vi "通道数对话框.vi"(8 "error in (no error)":errorcluster) -> (0 "error out":errorcluster)   [LabVIEW 2015]
uses:
  Global/SeverGlobal.vi
panel:
  in  "OK":bool
  in  "Channel count":enum16{"64X4", "128X4"}(ring)=enum."128X4"
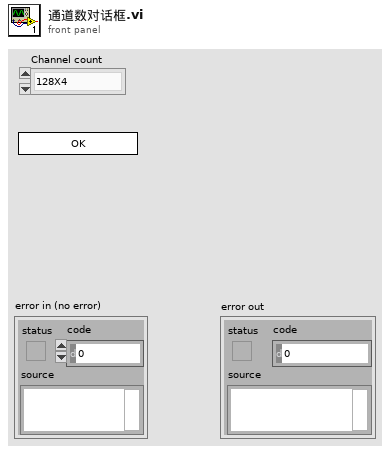
[diagram p1: front panel]
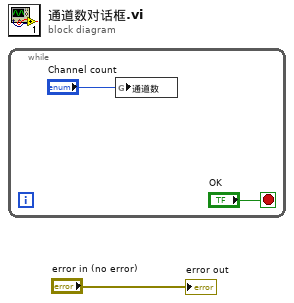
[diagram p0: block diagram]
diagram:
  n1 = while {
    stop <- "OK" stop-if-true
    n2 = global write "SeverGlobal.vi" "通道数"("Channel count") -> ()
  }
  "error out" <- "error in (no error)"
